vi "Key - String Write.vi"(8 "error in (no error)":errorcluster, 10 "String Ref in":refnum<vi>, 11 "Refnum in":T1) -> (0 "error out":errorcluster, 2 "spreadsheet string":string, 3 "Refnum out":T1)   [LabVIEW 2013]
uses:
  <vilib>/Utility/config.llb/Config Data RefNum.ctl
  <vilib>/Utility/config.llb/Write Key (String).vi
  <vilib>/Utility/config.llb/NI_LVConfig.lvlib
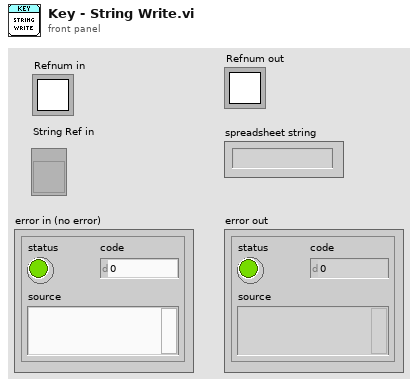
[diagram p1: front panel]
types:
  T1 = typedef "NI_LVConfig.lvlib/Config Data RefNum.ctl" = refnum<k1>
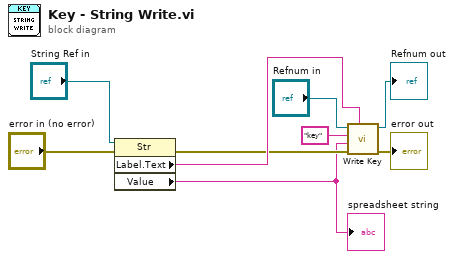
[diagram p0: block diagram]
diagram:
  n1 = property class="Str"(reference="String Ref in", error in="error in (no error)") -> (error out=w7:errorcluster, "Label.Text"=w8:string, "Value"=w1:string)  [unwired: 1 out]
  "spreadsheet string" <- w1
  n2 = call-poly <vilib>:"Write Key.vi"("section"=w8, "error in (no error)"=w7, "value"=w1, "key"="key" ("section"), "refnum"="Refnum in") -> ("error out"=→"error out":errorcluster, "refnum out"=→"Refnum out":T1)  [unwired: 4 in, 1 out]
